vi "Get Last Point.vi"(11 "Array":cluster{dbl, dbl, dbl}[](array[cluster])) -> (3 "Last Point":cluster{dbl, dbl, dbl})   [LabVIEW 2017]
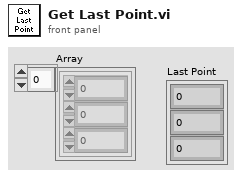
[diagram p1: front panel]
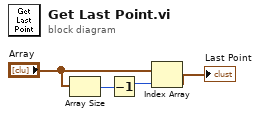
[diagram p0: block diagram]
diagram:
  n1 = Array Size(array="Array") -> (size(s)=w3:i32)
  n2 = Decrement(x=w3) -> (x-1=w4:i32)
  n3 = Index Array(array="Array", index=w4) -> (element=→"Last Point":cluster{dbl, dbl, dbl})
